vi "UTF-8 to Text (LabVIEW Path).vi"(8 "error in":errorcluster, 10 "Encoding (system default=-1)":i32=-1, 11 "UTF-8 Encoded Path":T1) -> (0 "error out":errorcluster, 3 "Path":path)   [LabVIEW 2020, in "G-Unicode.lvlib"]
uses:
  G-Unicode.lvlib
  Types/Encoded UTF-8 Path.ctl
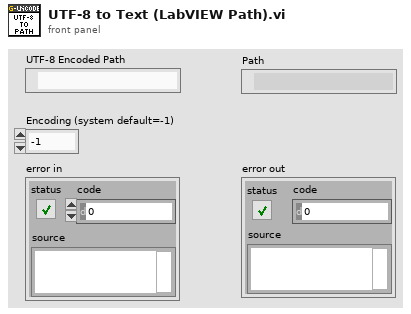
[diagram p1: front panel]
types:
  T1 = typedef "G-Unicode.lvlib/Encoded UTF-8 Path.ctl" = path
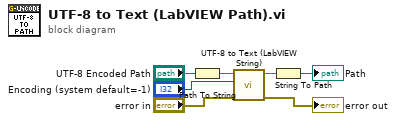
[diagram p0: block diagram]
diagram:
  n1 = Path To String(path="UTF-8 Encoded Path") -> (string=w3:string)
  n2 = call "UTF-8 to Text (LabVIEW String).vi"("error in"="error in", "Encoding (system default=-1)"="Encoding (system default=-1)", "UTF-8 Encoded String"=w3) -> ("error out"=→"error out":errorcluster, "String"=w2:string)  [unwired: 7 in]
  n3 = String To Path(string=w2) -> (path=→"Path":path)
